vi "Remove From Role Map.vi"(8 "error in (no error)":errorcluster, 10 "Name":string, 11 "Coffee Shop In":refnum<class "Coffee Shop.lvclass">) -> (0 "error out":errorcluster, 2 "Result Message":string, 3 "Coffee Shop Out":refnum<class "Coffee Shop.lvclass">)   [LabVIEW 2020, in "Coffee Shop.lvclass"]
uses:
  Coffee Shop.lvclass
  Coffee Shop.lvclass/Coffee Shop.ctl
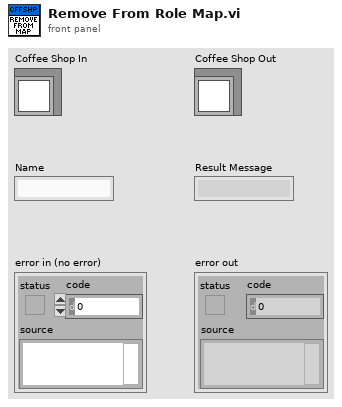
[diagram p1: front panel]
types:
  T1 = typedef "Coffee Shop.lvclass/Roles.ctl" = enum16{"Customer", "Barista", "Cashier"}
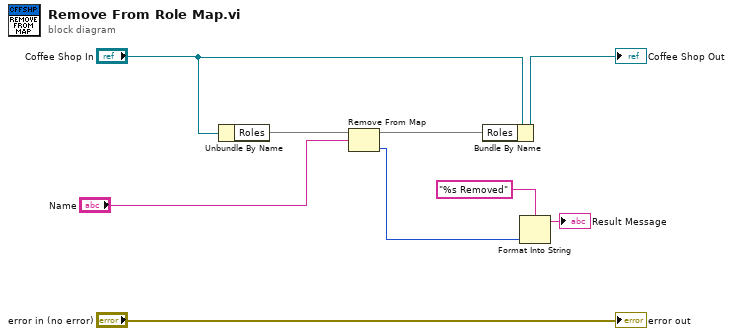
[diagram p0: block diagram]
diagram:
  n1 = Unbundle By Name("Coffee Shop In") -> ("Roles"=w6:map{string, T1})
  n2 = Remove From Map(10:"Name", 11:w6) -> (1:w3:T1, 3:w5:map{string, T1})  [unwired: 1 out]
  n3 = Bundle By Name(cluster="Coffee Shop In", "Roles"=w5) -> (→"Coffee Shop Out":refnum<class "Coffee Shop.lvclass">)
  n4 = Format Into String(format string="%s Removed", w3) -> (resulting string=→"Result Message":string)  [unwired: 2 in, 1 out]
  "error out" <- "error in (no error)"
